vi "Helper - Rounding Direction Chooser.vi"(6 "Buoy\nSide":enum16{"Starboard", "Port"}(ring), 7 "Starting location":T1 {"North" format="%#_10f"; "East" format="%#_8f"}, 8 "Point NORTH 2":dbl, 9 "Point EAST 2":dbl, 10 "Point NORTH":dbl, 11 "Point EAST":dbl) -> (0 "End Point NORTH":dbl, 1 "End Point EAST":dbl, 2 "Start Point NORTH":dbl, 3 "Start Point EAST":dbl)   [LabVIEW 2011]
doc: "This VI takes two previously created waypoints as input. Depending on the state of the ENUM variable (Starboard or Port) the attributes STARTPOINT and ENDPOINT are assigned to the two points."
uses:
  2 Typedefs/UTM Location.ctl
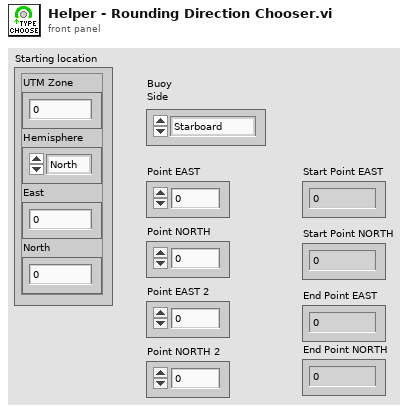
[diagram p1: front panel]
types:
  T1 = typedef "UTM Location.ctl" = cluster{"UTM Zone":dbl, "Hemisphere":enum16{"North", "South"}, "East":dbl, "North":dbl}
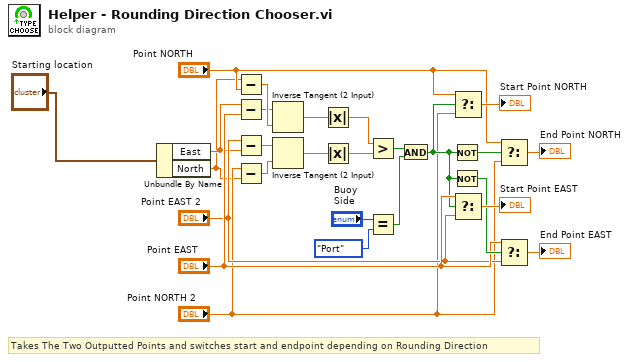
[diagram p0: block diagram]
diagram:
  # "Takes The Two Outputted Points and switches start and endpoint depending on Rounding Direction"
  n1 = Unbundle By Name("Starting location") -> ("East"=w4:dbl, "North"=w2:dbl)
  n2 = Subtract(x=w2, y="Point NORTH") -> (x-y=w24:dbl)
  n3 = Subtract(x=w4, y="Point EAST") -> (x-y=w23:dbl)
  n4 = Subtract(x="Point EAST 2", y=w4) -> (x-y=w22:dbl)
  n5 = Subtract(x="Point NORTH 2", y=w2) -> (x-y=w21:dbl)
  n6 = Inverse Tangent (2 Input)(1:w24, 2:w23) -> (0:w20:dbl)
  n7 = Inverse Tangent (2 Input)(1:w21, 2:w22) -> (0:w8:dbl)
  n8 = Absolute Value(x=w20) -> (abs(x)=w19:dbl)
  n9 = Absolute Value(x=w8) -> (abs(x)=w7:dbl)
  n10 = Greater?(x=w19, y=w7) -> (0:w18:bool)
  n11 = Equal?(x="Buoy\nSide", y=enum16{"Starboard", "Port"}."Port") -> (x = y?=w12:bool)
  n12 = And(x=w18, y=w12) -> (x .and. y?=w6:bool)
  n13 = Not(x=w6) -> (.not. x?=w16:bool)
  n14 = Not(x=w6) -> (.not. x?=w11:bool)
  n15 = Select(t="Point NORTH", s=w6, f="Point NORTH 2") -> (s? t:f=→"Start Point NORTH":dbl)
  n16 = Select(t="Point EAST", s=w6, f="Point EAST 2") -> (s? t:f=→"Start Point EAST":dbl)
  n17 = Select(t="Point NORTH", s=w16, f="Point NORTH 2") -> (s? t:f=→"End Point NORTH":dbl)
  n18 = Select(t="Point EAST", s=w11, f="Point EAST 2") -> (s? t:f=→"End Point EAST":dbl)
